vi "x_rotmatrix.vi"(1 "x-angle":dbl format="%.2f") -> (0 "x-matrix":dbl[][](array[numeric])=[[1.0, 0.0, 0.0, 0.0], [0.0, 1.0, -0.0, 0.0], [0.0, 0.0, 1.0, 0.0], [0.0, 0.0, 0.0, 1.0]] format="%.2f")   [LabVIEW 2011]
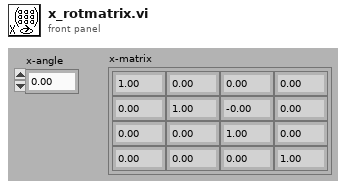
[diagram p1: front panel]
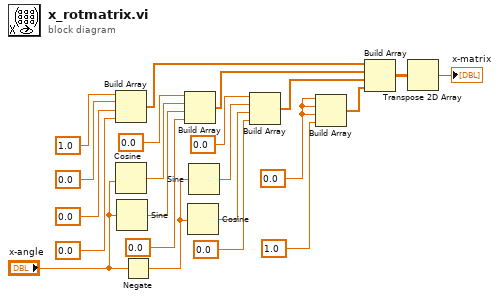
[diagram p0: block diagram]
diagram:
  w1 = 0.0
  n1 = Build Array(1.0, 0.0, 0.0, 0.0) -> (w20:dbl[])
  n2 = Cosine(x="x-angle") -> (cos(x)=w16:dbl)
  n3 = Sine(x="x-angle") -> (sin(x)=w17:dbl)
  n4 = Negate(x="x-angle") -> (-x=w13:dbl)
  n5 = Build Array(0.0, w16, w17, 0.0) -> (w21:dbl[])
  n6 = Cosine(x=w13) -> (cos(x)=w19:dbl)
  n7 = Sine(x=w13) -> (sin(x)=w18:dbl)
  n8 = Build Array(0.0, w18, w19, 0.0) -> (w22:dbl[])
  n9 = Build Array(w1, w1, w1, 1.0) -> (w6:dbl[])
  n10 = Build Array(w20, w21, w22, w6) -> (w11:dbl[][])
  n11 = Transpose 2D Array(2D array=w11) -> (transposed array=→"x-matrix":dbl[][])
